vi "Sample 4 - Async Waiting for Stop.vi"() -> ()   [LabVIEW 2016]
panel:
  in  "System Locator":string="usb:ix:0"
  in  "Delta Steps":i32[](array[numeric])=[50000, -100000, 200000, -400000]
  in  "stop":bool
  out "Error":errorcluster
  in  "Channel":u32=1
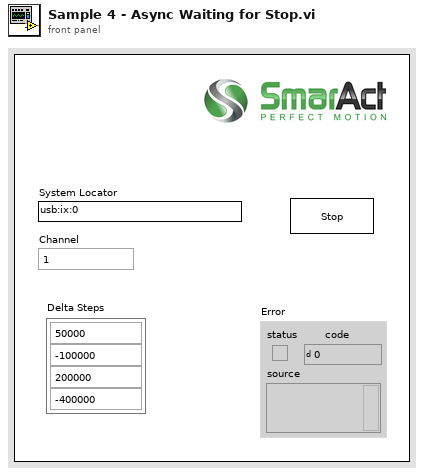
[diagram p1: front panel]
types:
  T1 = enum32{"SA_SENSOR_DISABLED", "SA_SENSOR_ENABLED", "SA_SENSOR_POWERSAVE"}
  T2 = enum32{"SA_UNBUFFERED_OUTPUT", "SA_BUFFERED_OUTPUT"}
  T3 = typedef "mcsPacket.ctl" = cluster{"packetType":enum32{"SA_NO PACKET_TYPE", "SA_ERROR_ PACKET_TYPE", "SA_POSITION PACKET_TYPE", "SA_COMPLETED PACKET_TYPE", "SA_STATUS PACKET_TYPE", "SA_ANGLE_PACKET_TYPE", "SA_VOLTAGE_LEVEL_PACKET_TYPE", "SA_SENSOR_TYPE_PACKET_TYPE", "SA_SENSOR_ENABLED_PACKET_TYPE", "SA_END_EFFECTOR_TYPE_PACKET_TYPE", "SA_GRIPPER_OPENING_PACKET_TYPE", "SA_FORCE_PACKET_TYPE", "SA_MOVE_SPEED_PACKET_TYPE", "SA_PHYSICAL_POSITION_KNOWN_PACKET_TYPE", "SA_POSITION_LIMIT_PACKET_TYPE", "SA_ANGLE_LIMIT_PACKET_TYPE", "SA_SAFE_DIRECTION_PACKET_TYPE", "SA_SCALE_PACKET_TYPE", "SA_MOVE_ACCELERATION_PACKET_TYPE", "SA_CHANNEL_PROPERTY_PACKET_TYPE", "SA_CAPTURE_BUFFER_PACKET_TYPE", "SA_TRIGGERED_PACKET_TYPE"}, "channelIndex":u32, "data1":u32, "data2":i32, "data3":i32, "data4":u32}
  T4 = enum32{"SA_NO PACKET_TYPE", "SA_ERROR_ PACKET_TYPE", "SA_POSITION PACKET_TYPE", "SA_COMPLETED PACKET_TYPE", "SA_STATUS PACKET_TYPE", "SA_ANGLE_PACKET_TYPE", "SA_VOLTAGE_LEVEL_PACKET_TYPE", "SA_SENSOR_TYPE_PACKET_TYPE", "SA_SENSOR_ENABLED_PACKET_TYPE", "SA_END_EFFECTOR_TYPE_PACKET_TYPE", "SA_GRIPPER_OPENING_PACKET_TYPE", "SA_FORCE_PACKET_TYPE", "SA_MOVE_SPEED_PACKET_TYPE", "SA_PHYSICAL_POSITION_KNOWN_PACKET_TYPE", "SA_POSITION_LIMIT_PACKET_TYPE", "SA_ANGLE_LIMIT_PACKET_TYPE", "SA_SAFE_DIRECTION_PACKET_TYPE", "SA_SCALE_PACKET_TYPE", "SA_MOVE_ACCELERATION_PACKET_TYPE", "SA_CHANNEL_PROPERTY_PACKET_TYPE", "SA_CAPTURE_BUFFER_PACKET_TYPE", "SA_TRIGGERED_PACKET_TYPE"}
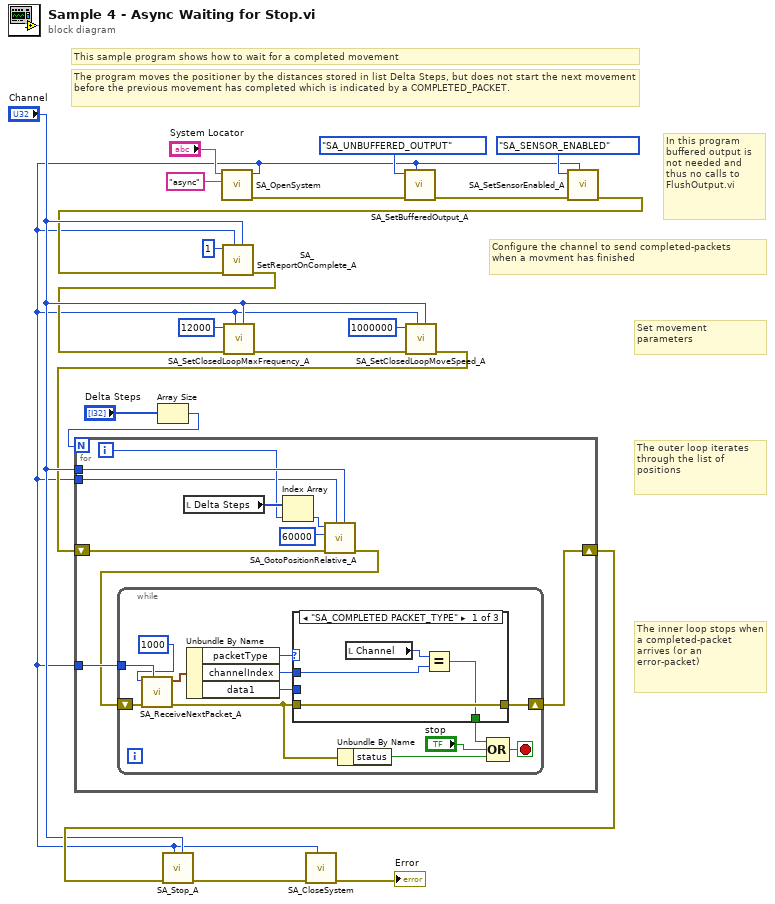
[diagram p0: block diagram]
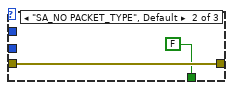
[diagram p2: hidden frame]
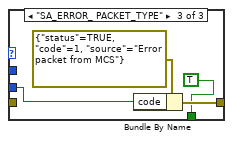
[diagram p3: hidden frame]
diagram:
  # "In this program buffered output is not needed and thus no calls to FlushOutput.vi"
  # "Set movement parameters"
  # "The program moves the positioner by the distances stored in list Delta Steps, but does not start the next movement before the previous movement has completed which is indicated by a COMPLETED_PACKET."
  # "The outer loop iterates through the list of positions"
  # "The inner loop stops when a completed-packet arrives (or an error-packet)"
  # "This sample program shows how to wait for a completed movement"
  # "Configure the channel to send completed-packets\nwhen a movment has finished"
  n1 = Array Size(array="Delta Steps") -> (size(s)=w15:i32)
  n2 = call <vilib>:"SA_OpenSystem.vi"("options"="async", "systemLocator"="System Locator") -> ("error out"=w20:errorcluster, "systemIndexOut"=w1:u32)  [unwired: 8 in]
  n3 = call <vilib>:"SA_SetBufferedOutput_A.vi"("systemIndex"=w1, "error in (no error)"=w20, "mode"=T2."SA_UNBUFFERED_OUTPUT") -> ("error out"=w7:errorcluster)  [unwired: 8 in]
  n4 = call <vilib>:"SA_SetSensorEnabled_A.vi"("systemIndex"=w1, "error in (no error)"=w7, "enabled"=T1."SA_SENSOR_ENABLED") -> ("error out"=w6:errorcluster)  [unwired: 8 in]
  n5 = call <vilib>:"SA_SetReportOnComplete_A.vi"("channelIndex"="Channel", "systemIndex"=w1, "error in (no error)"=w6, "report"=u32 1 ("systemIndex")) -> ("error out"=w8:errorcluster)  [unwired: 7 in]
  n6 = call <vilib>:"SA_SetClosedLoopMaxFrequency_A.vi"("channelIndex"="Channel", "systemIndex"=w1, "error in (no error)"=w8, "frequency"=u32 12000) -> ("error out"=w12:errorcluster)  [unwired: 7 in]
  n7 = call <vilib>:"SA_SetClosedLoopMoveSpeed_A.vi"("channelIndex"="Channel", "systemIndex"=w1, "error in (no error)"=w12, "speed"=u32 1000000) -> ("error out"=w4:errorcluster)  [unwired: 7 in]
  n8 = for {
    N: w15 -> [_]
    tunnel: w1 -> [w30]
    tunnel: "Channel" -> [w29]
    tunnel: w1 -> [w22]
    shift-right: [w26] -> w16
    shift-left: w4 -> [w28]
    i -> [w23]
    n9 = local read "Delta Steps"() -> (w24:i32[])
    n10 = Index Array(array=w24, index=w23) -> (element=w25:i32)
    n11 = call <vilib>:"SA_GotoPositionRelative_A.vi"("channelIndex"=w29, "systemIndex"=w22, "error in (no error)"=w28, "holdTime"=u32 60000, "diff"=w25) -> ("error out"=w21:errorcluster)  [unwired: 6 in]
    n12 = while {
      tunnel: w30 -> [w43]
      shift-right: [w39] -> w26
      shift-left: w21 -> [w40]
      stop <- w34 stop-if-true
      n13 = call <vilib>:"SA_ReceiveNextPacket_A.vi"("systemIndex"=w43, "error in (no error)"=w40, "timeout"=u32 1000) -> ("error out"=w35:errorcluster, "packet"=w41:T3)  [unwired: 7 in]
      n14 = Unbundle By Name(w41) -> ("packetType"=w36:T4, "channelIndex"=w37:u32, "data1"=w38:u32)
      n15 = case shown="\"SA_COMPLETED PACKET_TYPE\"" w36 {
        tunnel: w35 -> [w47 w49 _]
        tunnel: [w47 w49 w52] -> w39
        tunnel: w38 -> [_ _ w51]
        tunnel: [w46 FALSE TRUE] -> w33
        tunnel: w37 -> [w44 _ _]
        frame "SA_COMPLETED PACKET_TYPE" {
          n16 = local read "Channel"() -> (w45:u32)
          n17 = Equal?(x=w45, y=w44) -> (x = y?=w46:bool)
        }
        frame "SA_NO PACKET_TYPE", Default {
        }
        frame "SA_ERROR_ PACKET_TYPE" {
          n18 = Bundle By Name(cluster=errorcluster {"status"=TRUE, "code"=1, "source"="Error packet from MCS"} ("error out"), "code"=w51) -> (w52:errorcluster)
        }
      }
      n19 = Unbundle By Name(w35) -> ("status"=w31:bool)
      n20 = Compound Arithmetic op=OR(w33, "stop", w31) -> (w34:bool)
    }
  }
  n21 = call <vilib>:"SA_Stop_A.vi"("channelIndex"="Channel", "systemIndex"=w1, "error in (no error)"=w16) -> ("error out"=w5:errorcluster)  [unwired: 8 in]
  n22 = call <vilib>:"SA_CloseSystem.vi"("systemIndex"=w1, "error in (no error)"=w5) -> ("error out"=→"Error":errorcluster)  [unwired: 9 in]
